vi "Create.vi"(8 "error in (no error)":errorcluster, 10 "Element":refnum<class "Config Element.lvclass">) -> (0 "error out":errorcluster, 3 "Channel out":refnum<class "Channel.lvclass">)   [LabVIEW 2020, in "VolatusConfig.lvlib" / "Channel.lvclass"]
uses:
  Channel.lvclass
  Channel.lvclass/Channel.ctl
  lv-cdm/CDM-Config/Config Element/Config Element.lvclass
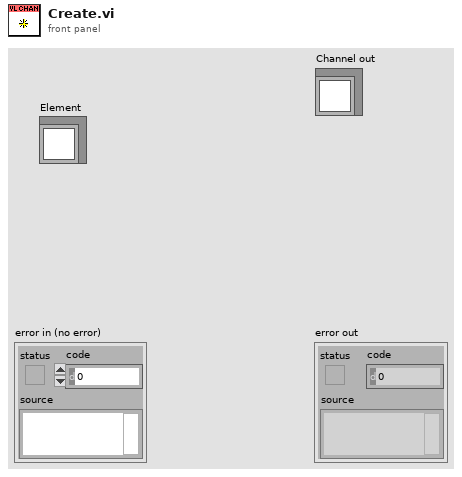
[diagram p1: front panel]
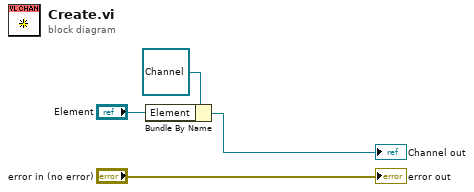
[diagram p0: block diagram]
diagram:
  n1 = Bundle By Name(cluster=refnum<class "Channel.lvclass"> refnum ("Channel in"), "Element"="Element") -> (→"Channel out":refnum<class "Channel.lvclass">)
  "error out" <- "error in (no error)"
